vi "Robot Main (robot acquires video).vi"() -> (0 "error out":errorcluster, 2 "Latest teleop command":T2)   [LabVIEW 2012]
doc: "Main VI that runs on the robot for teleoperation. This VI receives teleop commands from the host via UDP and sends video back to the host using network streams. This VI also acquires the image data from the robot's camera."
uses:
  ROV/Teleop command.ctl
  ROV/Safety commands.ctl
  <vilib>/userdefined/High Color/IMAQdx.ctl
  <vilib>/Platform/TimedLoop/XDataNode/timing_clust.ctl
  <vilib>/Platform/TimedLoop/XDataNode/nitl_modes.ctl
  <vilib>/Platform/TimedLoop/XDataNode/wakeup.ctl
  Robot globals (robot acquires video).vi
  <vilib>/Platform/TimedLoop/XDataNode/XDataNode.xnode
  <vilib>/vision/driver/NI_Vision_Acquisition_Software.lvlib
  <vilib>/Platform/TimedLoop/XDataNode/XDNodeRunTimeDep.lvlib
  ROV/ROV Host.lvclass
  <vilib>/robotics/Utilities/NI_Robotics Utilities.lvlib
panel:
  in  "Stop":bool
  out "Teleop command timed out":bool
  out "Safety commands":T1
  # "Before running this VI, select the robot's camera in this VI's block diagram at the initialization of the video acquisition (defaults to cam0)"
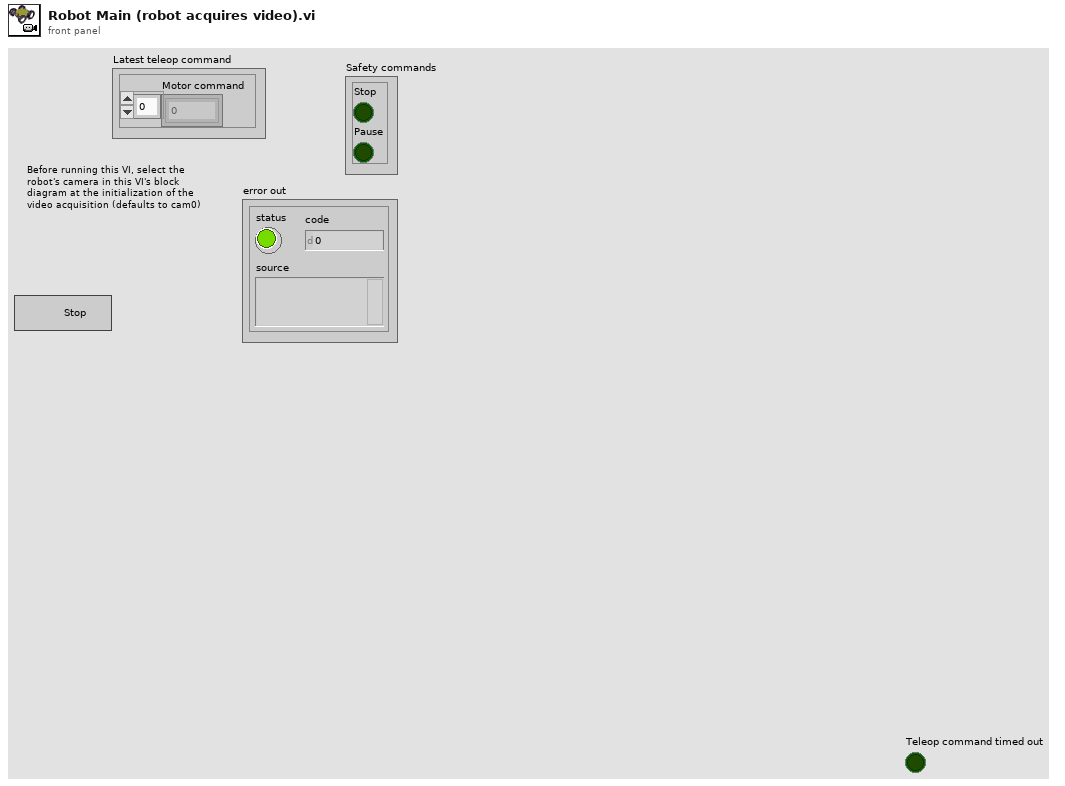
[diagram p1: front panel]
types:
  T1 = typedef "ROV Host.lvclass/Safety commands.ctl" = cluster{"Stop":bool, "Pause":bool}
  T2 = typedef "ROV Host.lvclass/Teleop command.ctl" = cluster{"Motor command":dbl[]}
  T3 = typedef "Image Type" = u32
  T4 = typedef "IMAQdx.ctl" = refnum<k21>
  T5 = typedef "IMAQ Image.ctl" = refnum<image>
  T6 = typedef "XDNodeRunTimeDep.lvlib/timing_clust.ctl" = cluster{"Expected End [f-1]":u64, "Actual End [f-1]":u64, "Finished Late? [f-1]":bool, "Expected End [i-1]":u64, "Actual End [i-1]":u64, "Finished Late? [i-1]":bool, "Expected Start [i]":u64, "Actual Start [i]":u64, "Expected Start [f]":u64, "Actual Start [f]":u64, "Source Name":string, "Structure Name":string, "Period":i64, "Deadline":i64, "Offset":i64, "Start":i64, "Priority":i32, "Timeout":i32, "Mode":T7, "Wakeup Reason":T8, "Error":errorcluster, "Source Type":string, "Secondary Source Type":string, "Global End Time":u64, "Global Start Time":u64, "Frame Duration":u64, "Iteration Duration":u64, "Assigned CPU":i32, "I/O Scan Engine Mode":u32}
  T7 = typedef "XDNodeRunTimeDep.lvlib/nitl_modes.ctl" = enum32{"No Change", "Process missed periods, maintain original phase", "Discard missed periods, maintain original phase", "Process missed periods, ignore original phase", "Discard missed periods, ignore original phase"}
  T8 = typedef "XDNodeRunTimeDep.lvlib/wakeup.ctl" = enum32{"Normal", "Aborted", "Asynchronous wakeup", "Timing source error", "Timed loop error", "Timeout"}
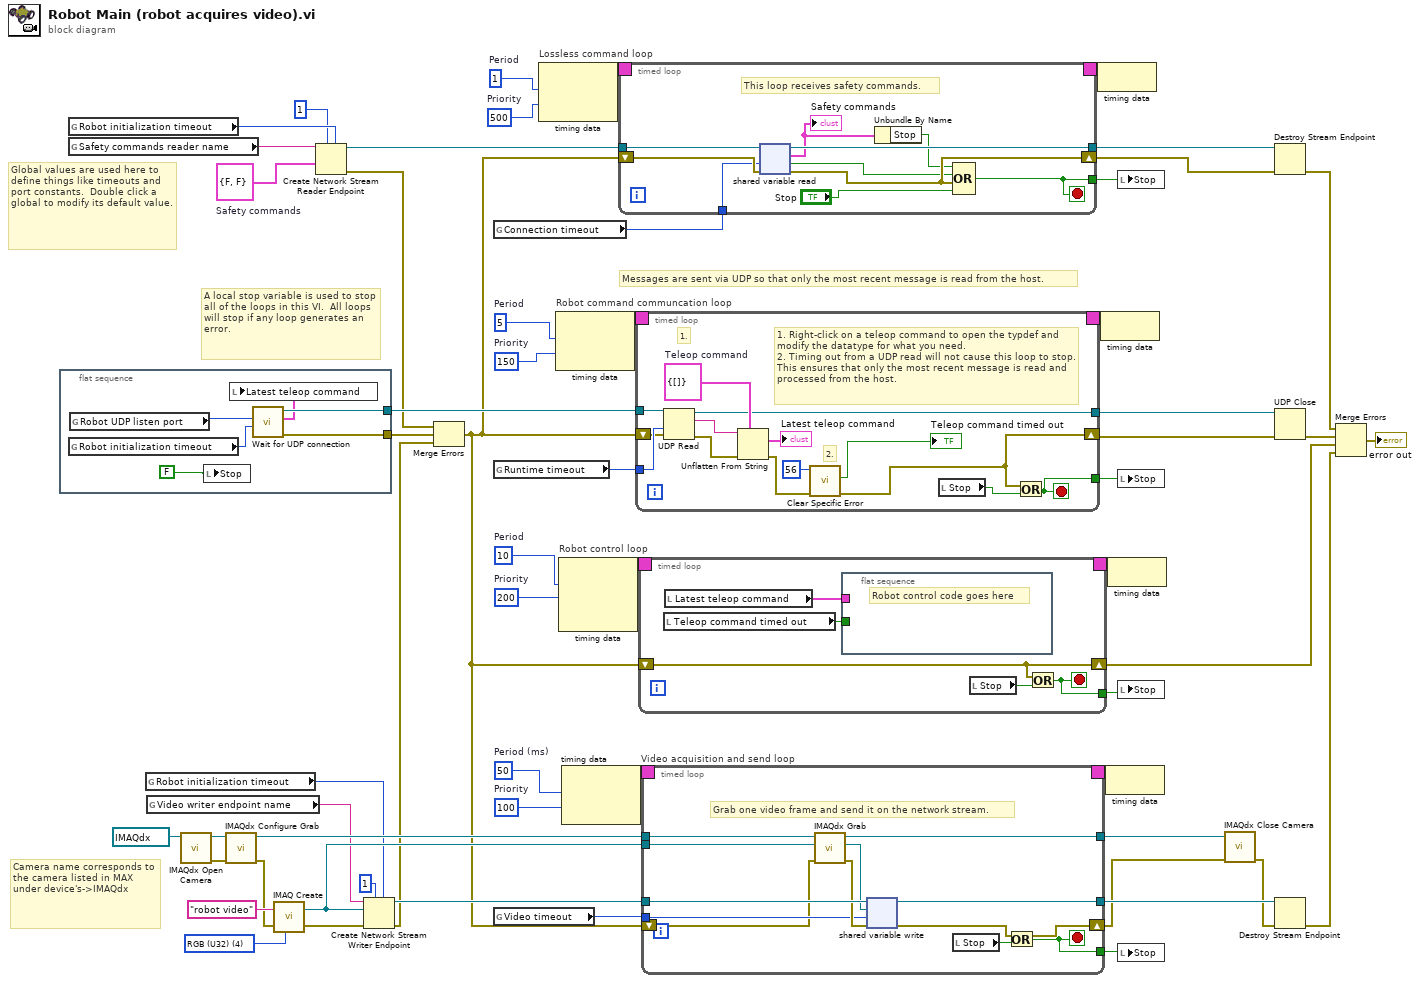
[diagram p0: block diagram]
diagram:
  w16 = T1 {"Stop"=FALSE, "Pause"=FALSE}  # Safety commands
  w9 = 500  # Priority
  w10 = i64 1  # Period
  w40 = 150  # Priority
  w39 = i64 5  # Period
  w43 = 200  # Priority
  w44 = i64 10  # Period
  w52 = T3 4 items=["Grayscale (U8)", "Grayscale (I16)", "Grayscale (SGL)", "Complex (CSG)", "RGB (U32)", "HSL (U32)", "RGB (U64)", "Grayscale (U16)"] ("Image Type")
  w55 = 100  # Priority
  w56 = i64 50  # Period (ms)
  # "Messages are sent via UDP so that only the most recent message is read from the host."
  # "Global values are used here to define things like timeouts and port constants.  Double click a global to modify its default value."
  # "A local stop variable is used to stop all of the loops in this VI.  All loops will stop if any loop generates an error."
  # "Camera name corresponds to the camera listed in MAX under device's->IMAQdx"
  n1 = flat-sequence {
    tunnel: [w65] -> w37
    tunnel: [w64] -> w36
    frame #0 {
      n2 = global read "Robot globals (robot acquires video).vi" "Robot initialization timeout"() -> (w62:i32)
      n3 = global read "Robot globals (robot acquires video).vi" "Robot UDP listen port"() -> (w63:u16)
      n4 = local write "Stop"(FALSE ("Stop")) -> ()
      n5 = call "Wait for UDP connection.vi"("Timeout (-1 never timeout)"=w62, "port (60200)"=w63) -> ("error out"=w65:errorcluster, "Initial teleop command"=w61:T2, "UDP Network Connection out"=w64:refnum<k16>)  [unwired: 7 in]
      n6 = local write "Latest teleop command"(w61) -> ()
    }
  }
  n7 = global read "Robot globals (robot acquires video).vi" "Robot initialization timeout"() -> (w13:i32)
  n8 = global read "Robot globals (robot acquires video).vi" "Safety commands reader name"() -> (w11:string)
  n9 = global read "Robot globals (robot acquires video).vi" "Robot initialization timeout"() -> (w4:i32)
  n10 = global read "Robot globals (robot acquires video).vi" "Video writer endpoint name"() -> (w26:string)
  n11 = call <vilib>:"IMAQdx Open Camera.vi"("Session In"=T4 "cam0") -> ("error out"=w30:errorcluster, "Session Out"=w29:T4)  [unwired: 9 in]
  n12 = call <vilib>:"IMAQdx Configure Grab.vi"("error in"=w30, "Session In"=w29) -> ("error out"=w28:errorcluster, "Session Out"=w27:T4)  [unwired: 8 in]
  n13 = call "IMAQ Create"("Image Name"="robot video", "Image Type"=w52, "error in (no error)"=w28) -> ("New Image"=w54:T5, "error out"=w38:errorcluster)  [unwired: 2 in]
  n14 = Create Network Stream Reader Endpoint(5:w13, 7:1 ("reader buffer size"), 9:w16, 11:w11) -> (0:w15:errorcluster, 3:w17:refnum<k21>)  [unwired: 3 in]
  n15 = Create Network Stream Writer Endpoint(5:w4, 7:1 ("writer buffer size"), 8:w38, 9:w54, 11:w26) -> (0:w24:errorcluster, 3:w50:refnum<k21>)  [unwired: 2 in]
  n16 = Merge Errors(w15, w37, w24) -> (w14:errorcluster)
  n17 = global read "Robot globals (robot acquires video).vi" "Connection timeout"() -> (w18:i32)
  n18 = global read "Robot globals (robot acquires video).vi" "Runtime timeout"() -> (w34:i32)
  n19 = global read "Robot globals (robot acquires video).vi" "Video timeout"() -> (w33:i32)
  n20 = node-c288(w10, w9) -> (w23:T6)
  n21 = node-c288(w39, w40) -> (w42:T6)
  n22 = node-c288(w44, w43) -> (w46:T6)  [unwired: 1 in]
  n23 = node-c288(w56, w55) -> (w58:T6)
  n24 = timed-loop "Lossless command loop" {
    timing: w23 -> [_]
    timing-out: [_] -> w22
    tunnel: w17 -> [w75]
    tunnel: [w74] -> w20
    tunnel: [w71] -> w8
    tunnel: w18 -> [w69]
    shift-right: [w70] -> w21
    shift-left: w14 -> [w73]
    stop <- w71 stop-if-true
    # "This loop receives safety commands."
    n25 = shared-variable-read(w75, w73, w69) -> (w74:refnum<k21>, w70:errorcluster, w67:bool, w72:T1)
    "Safety commands" <- w72
    n26 = Unbundle By Name(w72) -> ("Stop"=w68:bool)
    n27 = Compound Arithmetic op=OR(w68, w67, w70, "Stop") -> (w71:bool)
  }
  n28 = timed-loop "Robot command communcation loop" {
    timing: w42 -> [_]
    timing-out: [_] -> w41
    tunnel: w36 -> [w91]
    tunnel: [w86] -> w35
    tunnel: w34 -> [w85]
    tunnel: [w84] -> w5
    shift-right: [w80] -> w3
    shift-left: w14 -> [w83]
    stop <- w84 stop-if-true
    w87 = T2 {"Motor command"=[]}  # Teleop command
    # "2."
    # "1."
    # "1. Right-click on a teleop command to open the typdef and modify the datatype for what you need.\n2. Timing out from a UDP read will not cause this loop to stop. This ensures that only the most recent message is read and processed from the host."
    n29 = UDP Read(connection ID=w91, timeout ms (25000)=w85, 8:w83) -> (data out=w90:string, error out=w89:errorcluster, 3:w86:refnum<k16>)  [unwired: 1 in, 2 out]
    n30 = Unflatten From String(type=w87, binary string=w90, error in (no error)=w89) -> (value=→"Latest teleop command":T2, error out=w81:errorcluster)  [unwired: 2 in, 1 out]
    n31 = call <vilib>:"Clear Specific Error.vi"("error in (no error)"=w81, "code"=56) -> ("error out"=w80:errorcluster, "cleared?"=→"Teleop command timed out":bool)  [unwired: 7 in, 1 out]
    n32 = local read "Stop"() -> (w78:bool)
    n33 = Or(x=w80, y=w78) -> (x .or. y?=w84:bool)
  }
  n34 = timed-loop "Robot control loop" {
    timing: w46 -> [_]
    timing-out: [_] -> w45
    tunnel: [w98] -> w6
    shift-right: [w96] -> w2
    shift-left: w14 -> [w96]
    stop <- w98 stop-if-true
    n35 = local read "Teleop command timed out"() -> (w95:bool)
    n36 = local read "Latest teleop command"() -> (w97:T2)
    n37 = flat-sequence {
      tunnel: w97 -> [_]
      tunnel: w95 -> [_]
      frame #0 {
        # "Robot control code goes here"
      }
    }
    n38 = local read "Stop"() -> (w94:bool)
    n39 = Or(x=w96, y=w94) -> (x .or. y?=w98:bool)
  }
  n40 = timed-loop "Video acquisition and send loop" {
    timing: w58 -> [_]
    timing-out: [_] -> w57
    tunnel: w27 -> [w112]
    tunnel: w54 -> [w111]
    tunnel: w50 -> [w110]
    tunnel: [w107] -> w49
    tunnel: [w106] -> w48
    tunnel: w33 -> [w105]
    tunnel: [w104] -> w7
    shift-right: [w102] -> w1
    shift-left: w14 -> [w103]
    stop <- w104 stop-if-true
    # "Grab one video frame and send it on the network stream."
    n41 = call <vilib>:"IMAQdx Grab.vi"("error in"=w103, "Image In"=w111, "Session In"=w112) -> ("error out"=w108:errorcluster, "Image Out"=w109:T5, "Session Out"=w107:T4)  [unwired: 5 in, 1 out]
    n42 = shared-variable-write(w110, w108, w109, w105) -> (w106:refnum<k21>, w102:errorcluster)  [unwired: 1 out]
    n43 = local read "Stop"() -> (w101:bool)
    n44 = Or(x=w102, y=w101) -> (x .or. y?=w104:bool)
  }
  n45 = node-c288(w22) -> ()
  n46 = node-c288(w41) -> ()
  n47 = node-c288(w57) -> ()
  n48 = node-c288(w45) -> ()
  n49 = local write "Stop"(w8) -> ()
  n50 = local write "Stop"(w5) -> ()
  n51 = local write "Stop"(w6) -> ()
  n52 = local write "Stop"(w7) -> ()
  n53 = call <vilib>:"IMAQdx Close Camera.vi"("error in"=w1, "Session In"=w49) -> ("error out"=w47:errorcluster)  [unwired: 9 in]
  n54 = Destroy Stream Endpoint(8:w21, 11:w20) -> (0:w19:errorcluster)
  n55 = UDP Close(connection ID=w35, 8:w3) -> (error out=w32:errorcluster)  [unwired: 1 out]
  n56 = Destroy Stream Endpoint(8:w47, 11:w48) -> (0:w25:errorcluster)
  n57 = Merge Errors(w19, w32, w2, w25) -> (→"error out":errorcluster)
